vi "Unsaturate Commanded Motor Velocities.vi"(0 "motor command vel. (rad/s)":dbl[](array[numeric]), 1 "saturation rad/s":dbl) -> (2 "unsaturated motor command vel. (rad/s)":dbl[](array[numeric]))   [LabVIEW 2017]
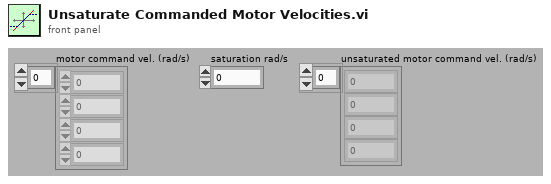
[diagram p1: front panel]
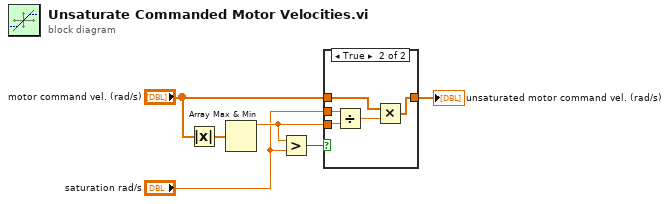
[diagram p0: block diagram]
diagram:
  n1 = Absolute Value(x="motor command vel. (rad/s)") -> (abs(x)=w6:dbl[])
  n2 = Array Max & Min(array=w6) -> (max value=w3:dbl)  [unwired: 3 out]
  n3 = Greater?(x=w3, y="saturation rad/s") -> (0:w5:bool)
  n4 = case shown="True" w5 {
    tunnel: "motor command vel. (rad/s)" -> [w7 w9]
    tunnel: w3 -> [_ w11]
    tunnel: "saturation rad/s" -> [_ w12]
    tunnel: [w7 w8] -> w1
    frame False {
    }
    frame True {
      n5 = Divide(x=w12, y=w11) -> (x/y=w10:dbl)
      n6 = Multiply(x=w9, y=w10) -> (x*y=w8:dbl[])
    }
  }
  "unsaturated motor command vel. (rad/s)" <- w1
